vi "LS336&Opticool_TempControl.vi"() -> ()   [LabVIEW 2024]
uses:
  Lake Shore 336/Lake Shore 336.lvlib
  <vilib>/Analysis/NI_AALBase.lvlib
  <vilib>/Analysis/baseanly.llb/Mean (DBL).vi
panel:
  in  "Ramp Rate (K/min)":dbl format="%.1f"
  in  "Setpoint Ramping \nEnable (F: Off)":bool
  in  "Power Up Enable":bool=TRUE
  in  "Mode (0:Off)":u16(ring)=1 items=["Off", "Closed Loop PID", "Zone", "Open Loop"]
  in  "Heater Resistance (1:25 Ohms)":u16(ring)=2 items=["25 Ohms"=1, "50 Ohms"=2]
  in  "Input (0:None)":u16(ring)=1 items=["None", "A", "B", "C", "D"]
  in  "Max Current (0:User Specified)":u16(ring) items=["User Specified", "0.707 A", "1.0 A", "1.141 A", "2.0 A"]
  in  "Heater Output (1:1)":u16(ring)=1 items=["1"=1, "2"=2]
  in  "VISA Model 336":refnum<visa-resource-name>
  out "Measuring (surface)":bool
  in  "Range (0:Off)":u16(ring)=1 items=["Off", "Low (On)", "Medium", "High"]
  in  "Temperature\nDifference":dbl
  in  "Crazy cooling\nMode":bool
  out "Opticool Temperature":dbl
  out "Opticool Field":dbl
  out "Opticool Temperature Status":i32(ring) items=["TemperatureUnknown"=0, "Stable"=1, "Tracking"=2, "Near"=5, "Chasing"=6, "Filling"=7, "Standby"=10, "Disabled"=13, "ImpedanceNotFunction"=14, "TempFailure"=15]
  out "Opticool Field Status":i32(ring) items=["MagnetUnknown"=0, "StablePersistent"=1, "WarmingSwitch"=2, "CoolingSwitch"=3, "StableDriven"=4, "Iterating"=5, "Charging"=6, "Discharging"=7, "CurrentError"=8, "MagnetFailure"=15]
  in  "Setfield (Oe)":dbl
  out "Measuring (Base)":bool
  in  "Opticool Address":string="127.0.0.1"
  in  "Setpoint (K)":dbl format="%.4f"
  out "Sensor Data":dbl format="%.4f"
  in  "Input (0:A)":u16(ring) items=["A", "B", "C", "D"]
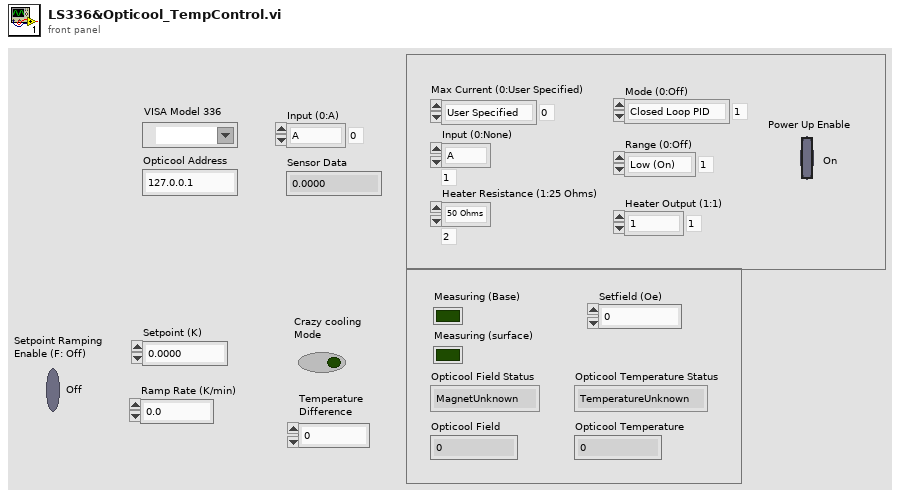
[diagram p1: front panel]
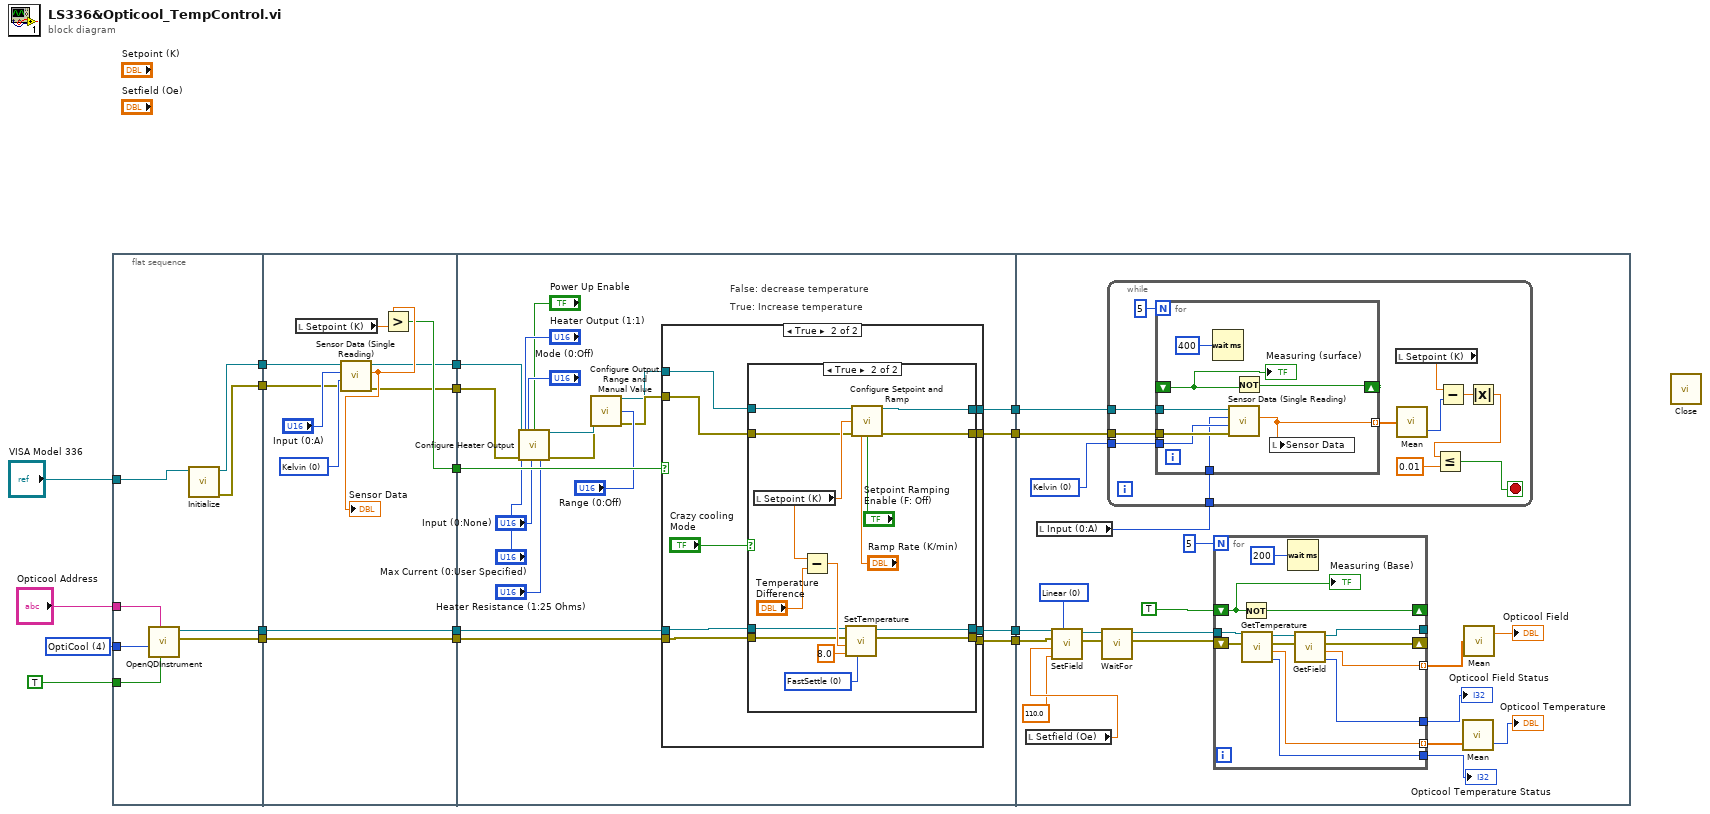
[diagram p0: block diagram]
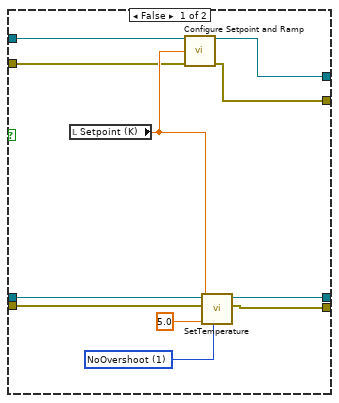
[diagram p2: hidden frame]
diagram:
  w13 = 4 items=["PPMS", "VersaLab", "DynaCool", "SVSM", "OptiCool"] ("InstrumentType")
  n1 = flat-sequence {
    tunnel: [w25] -> w16
    tunnel: TRUE ("Remote") -> [w24]
    tunnel: "Opticool Address" -> [w23]
    tunnel: w13 -> [w22]
    tunnel: [w21] -> w11
    tunnel: [w20] -> w7
    tunnel: [w19] -> w2
    tunnel: "VISA Model 336" -> [w18]
    tunnel: [w33] -> w17
    tunnel: w16 -> [w31]
    tunnel: [w30] -> w12
    tunnel: w11 -> [w30]
    tunnel: [w29] -> w8
    tunnel: w7 -> [w29]
    tunnel: [w28] -> w6
    tunnel: [w27] -> w5
    tunnel: w2 -> [w26]
    tunnel: w17 -> [w56]
    tunnel: w12 -> [w55]
    tunnel: [w54] -> w10
    tunnel: [w53] -> w9
    tunnel: w8 -> [w52]
    tunnel: w6 -> [w46]
    tunnel: w5 -> [w44]
    tunnel: [w48] -> w4
    tunnel: [w47] -> w3
    tunnel: w10 -> [w114]
    tunnel: w9 -> [w111]
    tunnel: w4 -> [w99]
    tunnel: w3 -> [w98]
    frame #0 {
      n2 = call "OpenQDInstrument.vi"("Remote"=w24, "IP Address"=w23, "InstrumentType"=w22) -> ("error out"=w20:errorcluster, "Instrument Ref"=w21:refnum<k24>)  [unwired: 5 in]
      n3 = call "Initialize.vi"("VISA resource name"=w18) -> ("error out"=w19:errorcluster, "VISA resource name out"=w25:refnum<visa-resource-name>)  [unwired: 9 in]
    }
    frame #1 {
      w32 = u16 0 items=["Kelvin", "Celsius", "Sensor Units"] ("Data Source (0:Kelvin)")
      n4 = local read "Setpoint (K)"() -> (w34:dbl)
      n5 = call "Sensor Data (Single Reading).vi"("error in (no error)"=w26, "Data Source (0:Kelvin)"=w32, "Input (0:A)"="Input (0:A)", "VISA resource name"=w31) -> ("error out"=w27:errorcluster, "Sensor Data"=w35:dbl, "VISA resource name out"=w28:refnum<visa-resource-name>)  [unwired: 5 in]
      "Sensor Data" <- w35
      n6 = Greater?(x=w35, y=w34) -> (0:w33:bool)
    }
    frame #2 {
      # "True: Increase temperature"
      # "False: decrease temperature"
      n7 = call "Configure Heater Output.vi"("VISA resource name"=w46, "Mode (0:Off)"="Mode (0:Off)", "Power Up Enable (F: Off)"="Power Up Enable", "Heater Output (1:1)"="Heater Output (1:1)", "Input (0:None)"="Input (0:None)", "Max Current (0:User Specified)"="Max Current (0:User Specified)", "error in (no error)"=w44, "Heater Resistance (1:25 Ohms)"="Heater Resistance (1:25 Ohms)") -> ("VISA resource name out"=w45:refnum<visa-resource-name>, "error out"=w43:errorcluster)  [unwired: 6 in]
      n8 = call "Configure Output Range and Manual Value.vi"("VISA resource name"=w45, "Range (0:Off)"="Range (0:Off)", "error in (no error)"=w43) -> ("VISA resource name out"=w49:refnum<visa-resource-name>, "error out"=w50:errorcluster)  [unwired: 11 in]
      n9 = case shown="True" w56 {
        tunnel: w55 -> [w64 w72]
        tunnel: [w63 w73] -> w54
        tunnel: [w62 w74] -> w53
        tunnel: w52 -> [w61 w75]
        tunnel: w50 -> [w60 w70]
        tunnel: w49 -> [w59 w71]
        tunnel: [w58 w69] -> w48
        tunnel: [w57 w68] -> w47
        frame False {
          w65 = 1 items=["FastSettle", "NoOvershoot"] ("Approach")
          n10 = local read "Setpoint (K)"() -> (w67:dbl)
          n11 = call "Configure Setpoint and Ramp.vi"("VISA resource name"=w59, "Setpoint (0.00000)"=w67, "error in (no error)"=w60) -> ("VISA resource name out"=w58:refnum<visa-resource-name>, "error out"=w57:errorcluster)  [unwired: 11 in]
          n12 = call "SetTemperature.vi"("Approach"=w65, "Rate"=5.0, "Temperature"=w67, "error in (no error)"=w61, "Instrument Ref In"=w64) -> ("error out"=w62:errorcluster, "Instrument Ref Out"=w63:refnum<k24>)  [unwired: 2 in, 1 out]
        }
        frame True {
          n13 = case shown="True" "Crazy cooling\nMode" {
            tunnel: w75 -> [w79 w92]
            tunnel: [w79 w91] -> w74
            tunnel: [w80 w90] -> w73
            tunnel: w72 -> [w80 w89]
            tunnel: w71 -> [w78 w86]
            tunnel: w70 -> [w77 w85]
            tunnel: [w78 w84] -> w69
            tunnel: [w77 w83] -> w68
            frame False {
            }
            frame True {
              w88 = 0 items=["FastSettle", "NoOvershoot"] ("Approach")
              n14 = local read "Setpoint (K)"() -> (w95:dbl)
              n15 = Subtract(x=w95, y="Temperature\nDifference") -> (x-y=w94:dbl)
              n16 = call "SetTemperature.vi"("Approach"=w88, "Rate"=8.0, "Temperature"=w94, "error in (no error)"=w92, "Instrument Ref In"=w89) -> ("error out"=w91:errorcluster, "Instrument Ref Out"=w90:refnum<k24>)  [unwired: 2 in, 1 out]
              n17 = call "Configure Setpoint and Ramp.vi"("VISA resource name"=w86, "Setpoint (0.00000)"=w95, "Setpoint Ramping \nEnable (F: Off)"="Setpoint Ramping \nEnable (F: Off)", "error in (no error)"=w85, "Ramp Rate (0.0)"="Ramp Rate (K/min)") -> ("VISA resource name out"=w84:refnum<visa-resource-name>, "error out"=w83:errorcluster)  [unwired: 9 in]
            }
          }
        }
      }
    }
    frame #3 {
      w97 = u16 0 items=["Kelvin", "Celsius", "Sensor Units"] ("Data Source (0:Kelvin)")
      w108 = 0 items=["Linear", "NoOvershoot", "Oscillate"] ("Approach")
      n18 = local read "Setfield (Oe)"() -> (w107:dbl)
      n19 = local read "Input (0:A)"() -> (w96:u16)
      n20 = call "SetField.vi"("Approach"=w108, "Rate"=110.0, "Field"=w107, "error in (no error)"=w111, "Instrument Ref In"=w114) -> ("error out"=w110:errorcluster, "Instrument Ref Out"=w113:refnum<k24>)  [unwired: 2 in, 1 out]
      n21 = call "WaitFor.vi"("error in (no error)"=w110, "Instrument Ref In"=w113) -> ("error out"=w109:errorcluster, "Instrument Ref Out"=w112:refnum<k24>)  [unwired: 8 in]
      n22 = while {
        tunnel: w99 -> [w128]
        tunnel: w98 -> [w127]
        tunnel: w97 -> [w126]
        tunnel: w96 -> [w117]
        stop <- w118 stop-if-true
        n23 = for {
          N: 5 -> [_]
          tunnel: w128 -> [w135]
          tunnel: w127 -> [w134]
          tunnel: w126 -> [w133]
          tunnel: [w132] -> w124 mode=indexing
          shift-right: [w131] -> _
          shift-left: _ -> [w130]
          tunnel: w117 -> [w129]
          n24 = Wait (ms)(milliseconds to wait=u32 400) -> ()  [unwired: 1 out]
          n25 = call "Sensor Data (Single Reading).vi"("error in (no error)"=w134, "Data Source (0:Kelvin)"=w133, "Input (0:A)"=w129, "VISA resource name"=w135) -> ("Sensor Data"=w132:dbl)  [unwired: 5 in, 2 out]
          n26 = Not(x=w130) -> (.not. x?=w131:bool)
          n27 = local write "Sensor Data"(w132) -> ()
          "Measuring (surface)" <- w130
        }
        n28 = local read "Setpoint (K)"() -> (w122:dbl)
        n29 = call-poly <vilib>:"Mean.vi"("X"=w124) -> ("error"=w123:i32)  [unwired: 1 out]
        n30 = Subtract(x=w122, y=w123) -> (x-y=w121:dbl)
        n31 = Absolute Value(x=w121) -> (abs(x)=w120:dbl)
        n32 = Less Or Equal?(x=w120, y=0.01) -> (x <= y?=w118:bool)
      }
      n33 = for {
        N: 5 -> [_]
        shift-right: [w149] -> _
        shift-left: TRUE -> [w137]
        shift-right: [w145] -> _
        shift-left: w109 -> [w147]
        tunnel: [w143] -> _
        tunnel: [w140] -> w105
        tunnel: [w139] -> w104
        tunnel: [w141] -> w103 mode=indexing
        tunnel: [w142] -> w101 mode=indexing
        tunnel: w112 -> [w138]
        n34 = Not(x=w137) -> (.not. x?=w149:bool)
        n35 = call "GetTemperature.vi"("error in (no error)"=w147, "Instrument Ref In"=w138) -> ("Temperature\nStatus"=w139:i32, "Temperature"=w142:dbl, "error out"=w146:errorcluster, "Instrument Ref Out"=w144:refnum<k24>)  [unwired: 3 in, 1 out]
        n36 = Wait (ms)(milliseconds to wait=u32 200) -> ()  [unwired: 1 out]
        n37 = call "GetField.vi"("error in (no error)"=w146, "Instrument Ref In"=w144) -> ("Field\nStatus"=w140:i32, "Field"=w141:dbl, "error out"=w145:errorcluster, "Instrument Ref Out"=w143:refnum<k24>)  [unwired: 3 in, 1 out]
        "Measuring (Base)" <- w137
      }
      "Opticool Field Status" <- w105
      "Opticool Temperature Status" <- w104
      n38 = call-poly <vilib>:"Mean.vi"("X"=w101) -> ("error"=→"Opticool Temperature":i32)  [unwired: 1 out]
      n39 = call-poly <vilib>:"Mean.vi"("X"=w103) -> ("mean"=→"Opticool Field":dbl)  [unwired: 1 out]
    }
  }
  n40 = call "Close.vi"() -> ()  [unwired: 11 in, 1 out]
